vi "Next_Folder.vi"(11 "Path in":path) -> (3 "Path out":path)   [LabVIEW 2012]
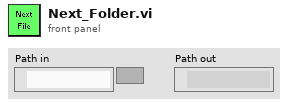
[diagram p1: front panel]
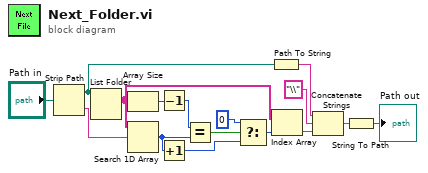
[diagram p0: block diagram]
diagram:
  n1 = Strip Path(path="Path in") -> (stripped path=w8:path, name=w3:string)
  n2 = List Folder(path=w8) -> (filenames=w11:string[])  [unwired: 3 in, 3 out]
  n3 = Array Size(array=w11) -> (size(s)=w4:i32)
  n4 = Search 1D Array(1D array=w11, element=w3) -> (index of element=w2:i32)  [unwired: 1 in]
  n5 = Decrement(x=w4) -> (x-1=w5:i32)
  n6 = Increment(x=w2) -> (x+1=w1:i32)
  n7 = Equal?(x=w5, y=w2) -> (x = y?=w14:bool)
  n8 = Select(t=0, s=w14, f=w1) -> (s? t:f=w16:i32)
  n9 = Path To String(path=w8) -> (string=w7:string)
  n10 = Index Array(array=w11, index=w16) -> (element=w6:string)
  n11 = Concatenate Strings(w7, "\\", w6) -> (w10:string)
  n12 = String To Path(string=w10) -> (path=→"Path out":path)
